vi "OptimizeMaxVel.vi"(9 "Settings in":T1, 10 "VISA resource name in":refnum<visa-resource-name>, 11 "TapeDrive in":refnum<class "TapeDrive.lvclass">) -> (1 "maxVel":dbl[](graph), 2 "Settings out":T1, 3 "TapeDrive out":refnum<class "TapeDrive.lvclass">)   [LabVIEW 2020, in "TapeDrive.lvclass"]
uses:
  TapeDrive.lvclass
  settings_TypDef.ctl
  shared/numericVariable_TypeDef.ctl
  shared/OnOffTypeDef.ctl
  Direction_TypDef.ctl
  Mode_TypDEf.ctl
  <vilib>/addons/_JKI.lib/Network_Streams_Connection.llb/PublicSettings.ctl
  <vilib>/Analysis/1siggen.llb/Ramp Pattern by Delta.vi
  <vilib>/Analysis/NI_AALBase.lvlib
  BaseDriver/BaseDriver.lvclass
  <vilib>/addons/_JKI.lib/Network_Streams_Connection.llb/NetworkConnection.lvclass
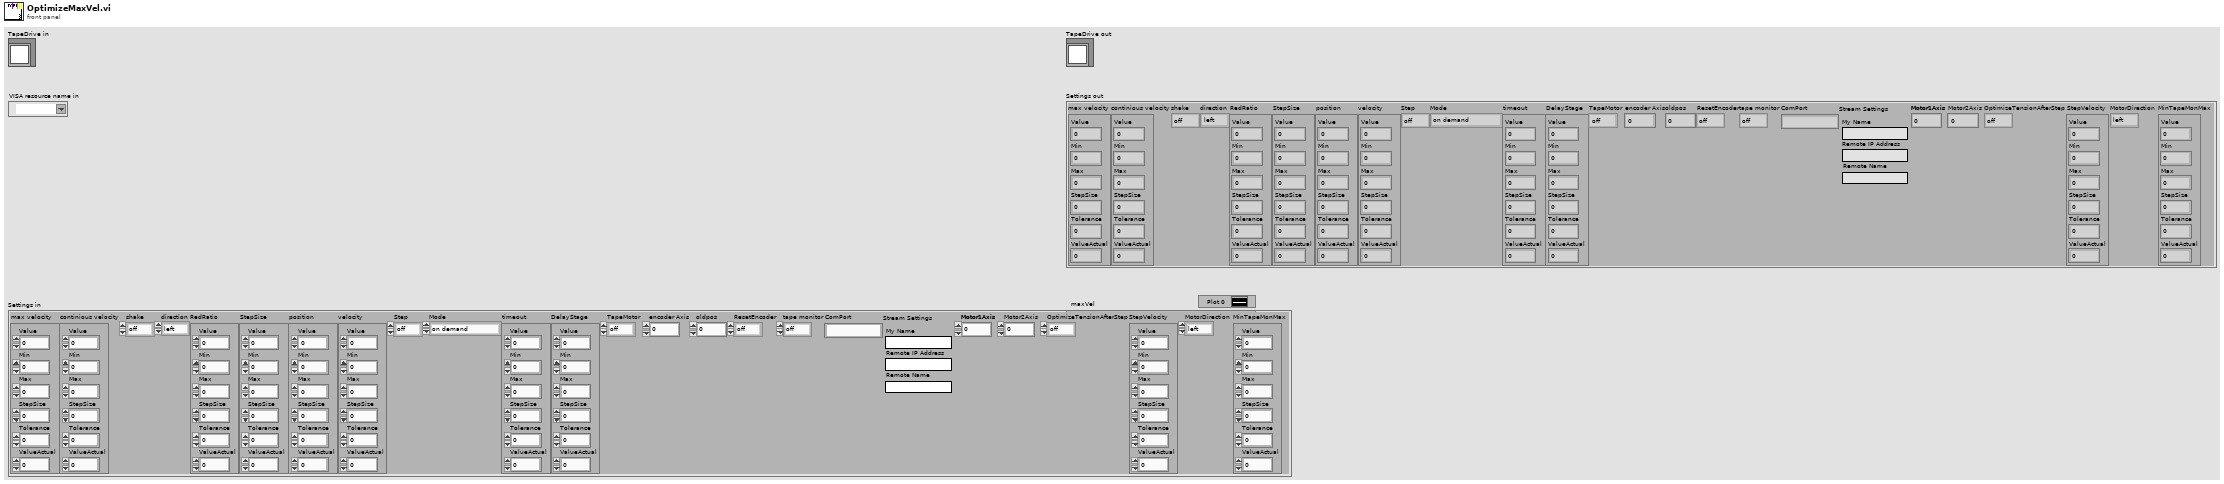
[diagram p1: front panel]
types:
  T1 = typedef "TapeDrive.lvclass/settings_TypDef.ctl" = cluster{"max velocity":T2, "continious velocity":T2, "shake":T3, "direction":T4, "RedRatio":T2, "StepSize":T2, "position":T2, "velocity":T2, "Step":T3, "Mode":T5, "timeout":T2, "DelayStage":T2, "TapeMotor":T3, "encoder Axis":i32, "oldpos":dbl, "ResetEncoder":T3, "tape monitor":T3, "ComPort":string, "Stream Settings":T6, "Motor1Axis":i32, "Motor2Axis":i32, "OptimizeTensionAfterStep":T3, "StepVelocity":T2, "MotorDirection":T4, "MinTapeMonMax":T2}
  T2 = typedef "BaseDriver.lvclass/numericVariable_TypeDef.ctl" = cluster{"Value":dbl, "Min":dbl, "Max":dbl, "StepSize":dbl, "Tolerance":dbl, "ValueActual":dbl}
  T3 = typedef "OnOffTypeDef.ctl" = enum16{"off", "on"}
  T4 = typedef "Direction_TypDef.ctl" = enum16{"left", "right"}
  T5 = typedef "Mode_TypDEf.ctl" = enum16{"on demand", "continuous", "scan"}
  T6 = typedef "NetworkConnection.lvclass/PublicSettings.ctl" = cluster{"My Name":string, "Remote IP Address":string, "Remote Name":string}
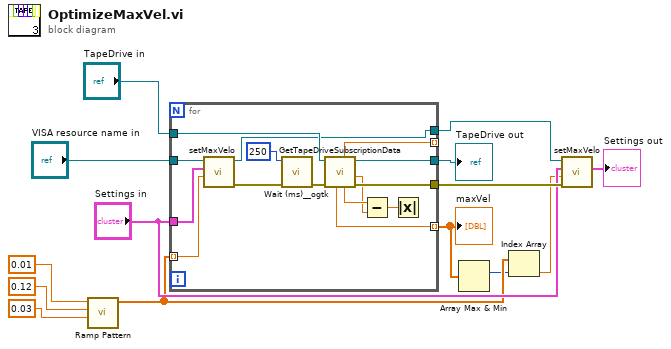
[diagram p0: block diagram]
diagram:
  n1 = call-poly <vilib>:"Ramp Pattern.vi"("start"=0.03, "end"=0.12, "delta"=0.01) -> ("Ramp Pattern"=w9:dbl[])  [unwired: 6 in, 2 out]
  n2 = for {
    tunnel: "VISA resource name in" -> [w29]
    tunnel: "Settings in" -> [w28]
    tunnel: w9 -> [w27] mode=indexing
    tunnel: "TapeDrive in" -> [w26]
    tunnel: [w25] -> w7
    tunnel: [w24] -> _ mode=indexing
    tunnel: [w15] -> w8 mode=indexing
    tunnel: [w20] -> w13
    tunnel: [w19] -> w14
    n3 = call "setMaxVelo.vi"("NewVal"=w27, "Settings"=w28, "VISA Refnum in"=w29) -> ("error out"=w21:errorcluster, "VISA Refnum out"=w20:refnum<visa-resource-name>)  [unwired: 5 in, 2 out]
    n4 = call <userlib>:"Wait (ms)__ogtk.vi"("error in (no error)"=w21, "milliseconds to wait"=u32 250) -> ("error out"=w23:errorcluster)  [unwired: 8 in, 1 out]
    n5 = call "GetTapeDriveSubscriptionData.vi"("error in (no error)"=w23, "TapeDrive in"=w26) -> ("error out"=w19:errorcluster, "TapeMonTargetY"=w17:dbl, "TapeDrive in 2"=w25:refnum<class "TapeDrive.lvclass">, "TapeMonCentroidY"=w18:dbl, "TapeMonCentroidX"=w24:dbl, "TapeMonMaxCounts"=w15:dbl)  [unwired: 3 in, 1 out]
    n6 = Subtract(x=w18, y=w17) -> (x-y=w16:dbl)
    n7 = Absolute Value(x=w16) -> ()  [unwired: 1 out]
  }
  "maxVel" <- w8
  "TapeDrive out" <- w7
  n8 = Array Max & Min(array=w8) -> (max index (indices)=w1:i32)  [unwired: 3 out]
  n9 = Index Array(array=w9, index=w1) -> (element=w10:dbl)
  n10 = call "setMaxVelo.vi"("error in (no error)"=w14, "NewVal"=w10, "Settings"="Settings in", "VISA Refnum in"=w13) -> ("Settings"=→"Settings out":T1)  [unwired: 4 in, 3 out]
